vi "dfd_Check Integer Delay.vi"(8 "error in (no error)":errorcluster, 10 "delay in":i32) -> (0 "error out":errorcluster, 2 "delay out":i32)   [LabVIEW 2017, in "NI_DigFilter_Process.lvlib"]
uses:
  <vilib>/addons/Digital Filter Design/NI_DigFilter_Process.lvlib
  <vilib>/addons/Digital Filter Design/_Misc.llb/dfd_Error Handlers (Single).vi
  <vilib>/addons/Digital Filter Design/NI_DigFilterLicensed.lvlib
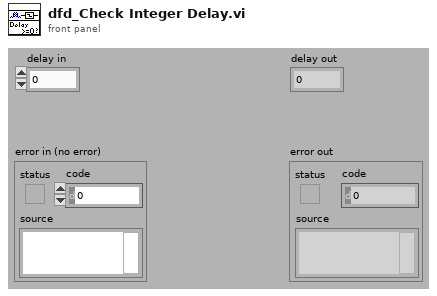
[diagram p1: front panel]
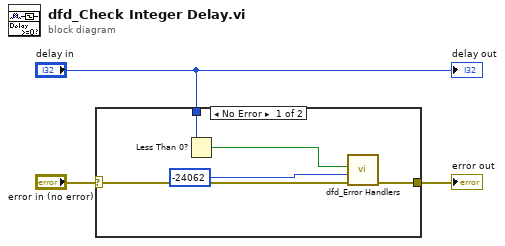
[diagram p0: block diagram]
diagram:
  n1 = case shown="No Error" "error in (no error)" {
    selector: "error in (no error)" -> [w7 w9]
    tunnel: [w4 w9] -> w2
    tunnel: "delay in" -> [w8 _]
    frame No Error {
      n2 = Less Than 0?(x=w8) -> (x < 0?=w5:bool)
      n3 = call-poly <vilib>:"dfd_Error Handlers.vi"("error in (no error)"=w7, "error code"=-24062 ("ERR_DELAY_LT_ZERO"), "condition failed?"=w5) -> ("error out"=w4:errorcluster)  [unwired: 8 out]
    }
    frame Error {
    }
  }
  "error out" <- w2
  "delay out" <- "delay in"
